vi "Valid.vi"(8 "error in (no error)":errorcluster, 11 "ColumnPanel in":refnum<class "ColumnPanel.lvclass">) -> (0 "error out":errorcluster, 1 "Issues":string[](array[string]), 2 "Valid?":bool)   [LabVIEW 2020, in "Conditum-Tools.lvlib" / "ColumnPanel.lvclass"]
uses:
  ColumnPanel.lvclass
  ColumnPanel.lvclass/ColumnPanel.ctl
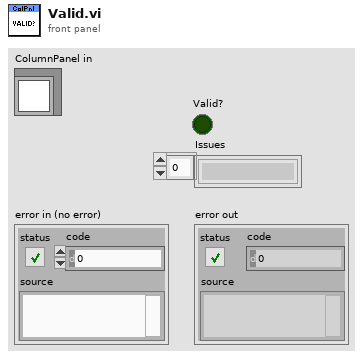
[diagram p1: front panel]
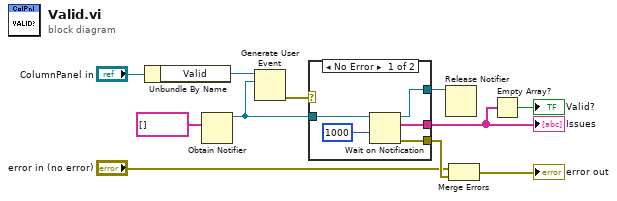
[diagram p0: block diagram]
diagram:
  n1 = Unbundle By Name("ColumnPanel in") -> ("Valid"=w11:refnum<user-event>)
  n2 = Obtain Notifier(notification data type=string[] []) -> (notifier out=w10:refnum<notifier>)  [unwired: 3 in, 2 out]
  n3 = Generate User Event(user event=w11, event data cluster=w10) -> (error out=w9:errorcluster)  [unwired: 2 in, 1 out]
  n4 = case shown="No Error" w9 {
    selector: w9 -> [_ w17]
    tunnel: w10 -> [w16 w18]
    tunnel: [w14 _] -> w4
    tunnel: [w13 w18] -> w8
    tunnel: [w12 w17] -> w7
    frame No Error {
      n5 = Wait on Notification(notifier=w16, timeout in ms (-1)=1000) -> (notifier out=w13:refnum<notifier>, notification=w14:string[], error out=w12:errorcluster)  [unwired: 2 in, 1 out]
    }
    frame Error {
    }
  }
  "Issues" <- w4
  n6 = Release Notifier(notifier=w8) -> ()  [unwired: 2 in, 3 out]
  n7 = Merge Errors("error in (no error)", w7) -> (→"error out":errorcluster)
  n8 = Empty Array?(array=w4) -> (empty?=→"Valid?":bool)
